vi "Read Settings File Name (SubVI).vi"() -> (3 "Settings File Name":path)   [LabVIEW 2020]
uses:
  <vilib>/Utility/config.llb/Read Key (String).vi
  <vilib>/Utility/config.llb/Write Key (String).vi
  <vilib>/Utility/config.llb/NI_LVConfig.lvlib
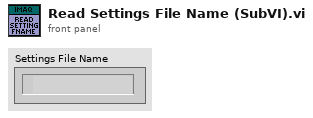
[diagram p1: front panel]
types:
  T1 = typedef "NI_LVConfig.lvlib/Config Data RefNum.ctl" = refnum<k1>
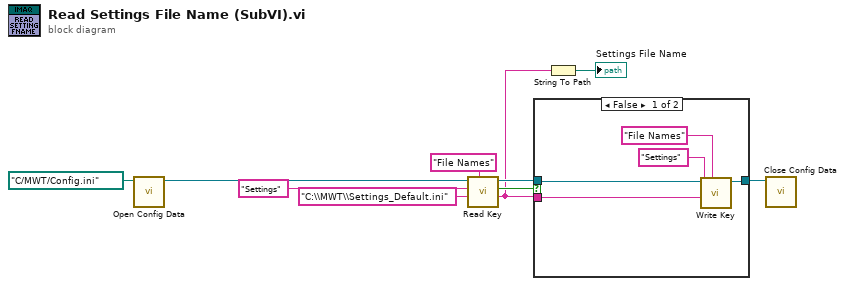
[diagram p0: block diagram]
diagram:
  n1 = call <vilib>:"Open Config Data.vi"("configuration file path"=path "C:/MWT/Config.ini") -> ("refnum"=w8:T1)  [unwired: 8 in, 2 out]
  n2 = call-poly <vilib>:"Read Key.vi"("section"="File Names", "default value"="C:\\MWT\\Settings_Default.ini", "key"="Settings" ("section"), "refnum"=w8) -> ("value"=w3:string, "found?"=w6:bool, "refnum out"=w5:T1)  [unwired: 4 in, 1 out]
  n3 = case shown="False" w6 {
    tunnel: w5 -> [w13 w16]
    tunnel: [w12 w16] -> w4
    tunnel: w3 -> [w11 _]
    frame False {
      n4 = call-poly <vilib>:"Write Key.vi"("section"="File Names", "value"=w11, "key"="Settings" ("section"), "refnum"=w13) -> ("refnum out"=w12:T1)  [unwired: 5 in, 2 out]
    }
    frame True {
    }
  }
  n5 = String To Path(string=w3) -> (path=→"Settings File Name":path)
  n6 = call <vilib>:"Close Config Data.vi"("refnum"=w4) -> ()  [unwired: 9 in, 2 out]
